vi "ble_discover_handle_table.vi"(6 "Connection Status":T1={"MAC Address"="", "cnx handle"=0, "cnx flags"=0, "Address Type"=125, "Connection Interval (ms)"=125, "Timeout(ms)"=125, "Latency"=0, "bonding handle"=0} {"Address Type" items=["Public", "Random"]}, 8 "error in (no error)":errorcluster, 11 "COM Bluegiga in":refnum<visa-resource-name>) -> (0 "error out":errorcluster, 2 "Handle table":string[][](array[string]), 3 "COM Bluegiga out":refnum<visa-resource-name>)   [LabVIEW 2015]
uses:
  type_def/connection_status_bundle.ctl
  type_def/address_type.ctl
panel:
  out "General Settings:Timeout Value":u32
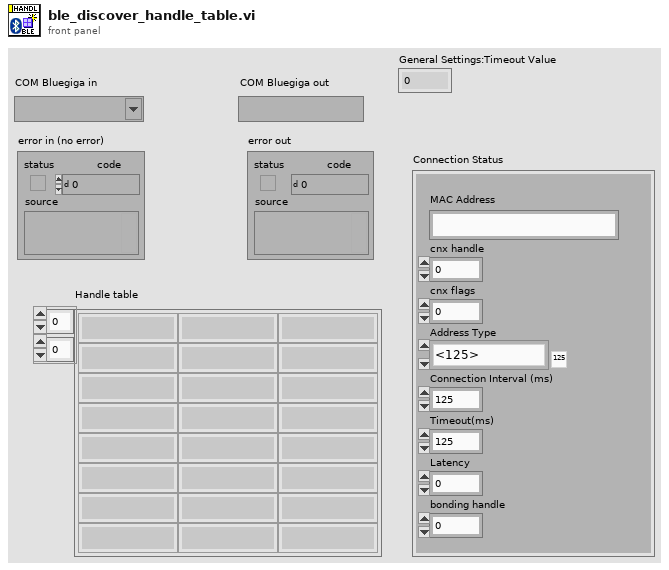
[diagram p1: front panel]
types:
  T1 = typedef "connection_status_bundle.ctl" = cluster{"MAC Address":string, "cnx handle":u8, "cnx flags":u8, "Address Type":T2, "Connection Interval (ms)":u16, "Timeout(ms)":u16, "Latency":u16, "bonding handle":u8}
  T2 = typedef "address_type.ctl" = u8
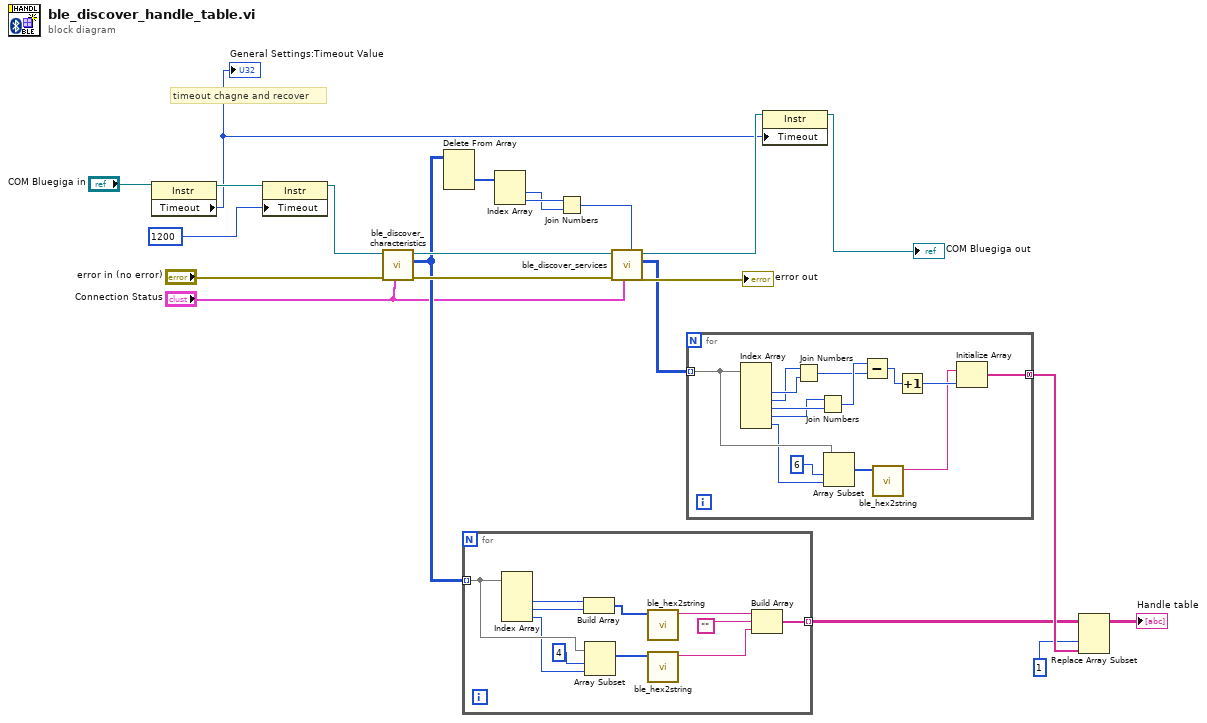
[diagram p0: block diagram]
diagram:
  # "timeout chagne and recover"
  n1 = property class="Instr"(reference="COM Bluegiga in") -> (reference out=w6:refnum<visa-resource-name>, "Timeout"=w1:u32)  [unwired: 1 in, 1 out]
  "General Settings:Timeout Value" <- w1
  n2 = property class="Instr"(reference=w6, "Timeout"=u32 1200 ("General Settings:Timeout Value")) -> (reference out=w4:refnum<visa-resource-name>)  [unwired: 1 in, 1 out]
  n3 = call "ble_discover_characteristics.vi"("Connection Status"="Connection Status", "error in (no error)"="error in (no error)", "COM Bluegiga in"=w4) -> ("error out"=w20:errorcluster, "characteristics_info"=w9:u8[][], "COM Bluegiga out"=w21:refnum<visa-resource-name>)  [unwired: 6 in]
  n4 = Delete From Array(array=w9) -> (deleted portion=w18:u8[])  [unwired: 3 in, 1 out]
  n5 = for {
    tunnel: w9 -> [w33] mode=indexing
    tunnel: [w31] -> w13 mode=indexing
    n6 = Index Array(array=w33) -> (element #2=w28:u8, element #3=w29:u8, element #4=w30:u8)  [unwired: 4 in, 1 out]
    n7 = Build Array(w28, w29) -> (w24:u8[])
    n8 = Array Subset(array=w33, index=4, length=w30) -> (w25:u8[])
    n9 = call "ble_hex2string.vi"("Byte Array IN (index0 LS byte)"=w24) -> ("HEX string OUT"=w23:string)  [unwired: 10 in]
    n10 = call "ble_hex2string.vi"("Byte Array IN (index0 LS byte)"=w25) -> ("HEX string OUT"=w26:string)  [unwired: 10 in]
    n11 = Build Array(w23, "", w26) -> (w31:string[])
  }
  n12 = Index Array(array=w18) -> (element #1=w16:u8, element #2=w17:u8)  [unwired: 2 in]
  n13 = Join Numbers(hi=w17, lo=w16) -> ((hi.lo)=w15:u16)
  n14 = call "ble_discover_services.vi"("Last Handle Number (0xFFFF)"=w15, "Connection Status"="Connection Status", "error in (no error)"=w20, "COM Bluegiga in"=w21) -> ("error out"=→"error out":errorcluster, "service_info"=w10:u8[][], "COM Bluegiga out"=w3:refnum<visa-resource-name>)  [unwired: 5 in]
  n15 = for {
    tunnel: w10 -> [w46] mode=indexing
    tunnel: [w42] -> w14 mode=concatenating
    n16 = Index Array(array=w46) -> (element #2=w37:u8, element #3=w36:u8, element #4=w35:u8, element #5=w34:u8, element #6=w45:u8)  [unwired: 6 in, 1 out]
    n17 = Join Numbers(hi=w36, lo=w37) -> ((hi.lo)=w40:u16)
    n18 = Join Numbers(hi=w34, lo=w35) -> ((hi.lo)=w41:u16)
    n19 = Array Subset(array=w46, index=6, length=w45) -> (w39:u8[])
    n20 = Subtract(x=w41, y=w40) -> (x-y=w47:u16)
    n21 = call "ble_hex2string.vi"("Byte Array IN (index0 LS byte)"=w39) -> ("HEX string OUT"=w38:string)  [unwired: 10 in]
    n22 = Increment(x=w47) -> (x+1=w43:u16)
    n23 = Initialize Array(w38, w43) -> (w42:string[])
  }
  n24 = property class="Instr"(reference=w3, "Timeout"=w1) -> (reference out=→"COM Bluegiga out":refnum<visa-resource-name>)  [unwired: 1 in, 1 out]
  n25 = Replace Array Subset(array=w13, new element=w14, index (col)=1 ("disabled index (col)")) -> (→"Handle table":string[][])  [unwired: 1 in]
